vi "Configurator.vi"(9 "CDependencyInspector in":refnum<class "CDependencyInspection.lvclass">, 11 "UIManager in":refnum<class "UIManager.lvclass">) -> (3 "UIManager out":refnum<class "UIManager.lvclass">)   [LabVIEW 2020, in "UserInterface.lvlib" / "UIManager.lvclass"]
uses:
  UIManager/UIManager.lvclass
  DependencyInspection/CItemMatch/TypeDefs/Field.ctl
  DependencyInspection/CItemMatch/TypeDefs/ComparisonType.ctl
  DependencyInspection/CDependencyInspector/CDependencyInspection.lvclass
  ExtensionInterfaces/IConfigurationPage/Event_ParametersRef.ctl
  ExtensionInterfaces/IConfigurationPage/Event_Parameters.ctl
  DependencyInspection/CDependencyInspector/Options.ctl
  DependencyInspection/CDependencyInspector/Options_Export.ctl
  DependencyInspection/CDependencyInspector/Options_Filter.ctl
  DependencyInspection/CItemMatch/CItemMatch.lvclass
  ExtensionInterfaces/IConfigurationPage/IConfigurationPage.lvclass
panel:
  in  "Tab Control":T1(tab)
  in  "Target filter":T4
  in  "Source filter":T4
  in  "Circular deps":bool
  in  "Top level only":bool
  in  "Tests into a separate group":bool
  in  "Path to Check":path
  in  "Exclude instances":bool=TRUE
  in  "Exclude external":bool=TRUE
  in  "Root Path":path
  in  "AND Condition?":bool
  in  "Rules parsers":string(combo)
  in  "Export Rules":bool=TRUE
  in  "Export Dependencies":bool=TRUE
  in  "Exporters":string(combo)
  in  "Export Invalid Dependencies":bool=TRUE
  in  "Export Concessions":bool=TRUE
  in  "Export Undeclared":bool=TRUE
  out "Results":string[][](table)
  in  "Close":bool
  in  "Run":bool
  # "Options"
  # "(780 x 230)"
  # "Options"
  # "(780 x 155)"
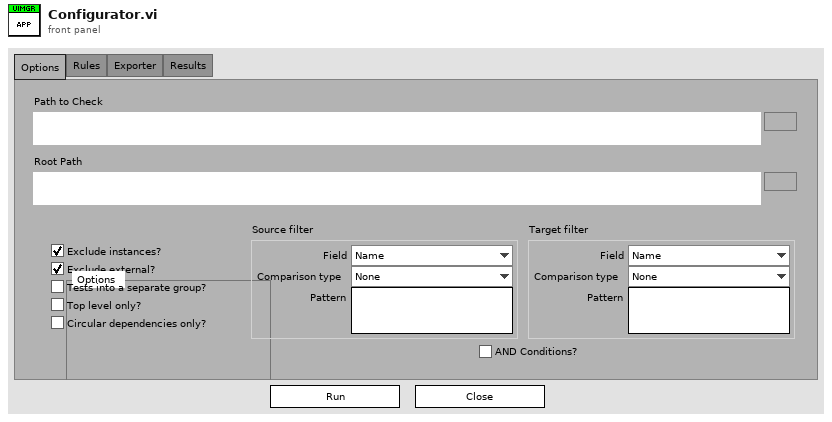
[diagram p1: front panel]
types:
  T1 = enum32{"Options", "Rules", "Exporter", "Results"}
  T2 = typedef "DependencyInspection.lvlib/CItemMatch.lvclass/Field.ctl" = enum16{"Name", "Qualified name", "Path"}
  T3 = typedef "DependencyInspection.lvlib/CItemMatch.lvclass/ComparisonType.ctl" = enum16{"None", "Ends with", "Equals", "Not equal", "Starts with", "Contains", "Matches pattern"}
  T4 = cluster{"Field":T2, "Comparison type":T3, "Pattern":string}
  T5 = typedef "ExtensionInterfaces.lvlib/IConfigurationPage.lvclass/Event_ParametersRef.ctl" = refnum<user-event>
  T6 = typedef "DependencyInspection.lvlib/CDependencyInspection.lvclass/Options.ctl" = cluster{"exclude instances?":bool, "exclude external? (T)":bool, "separate tests?":bool, "top level results only?":bool, "Export options":T7, "Filter options":T8, "quiet?":bool}
  T7 = typedef "DependencyInspection.lvlib/CDependencyInspection.lvclass/Options_Export.ctl" = cluster{"Export rules":bool, "Export dependencies":bool, "Export invalid dependencies":bool, "Export concessions":bool, "Export undeclared":bool}
  T8 = typedef "DependencyInspection.lvlib/CDependencyInspection.lvclass/Options_Filter.ctl" = cluster{"Source filter":refnum<class "CItemMatch.lvclass">, "Target filter":refnum<class "CItemMatch.lvclass">, "AND Condition?":bool}
  T9 = typedef "UserInterface.lvlib/UIManager.lvclass/subReferenceData.ctl" = cluster{"VI Ref":refnum<vi>, "Stop":refnum<user-event>, "Parameters":refnum<user-event>}
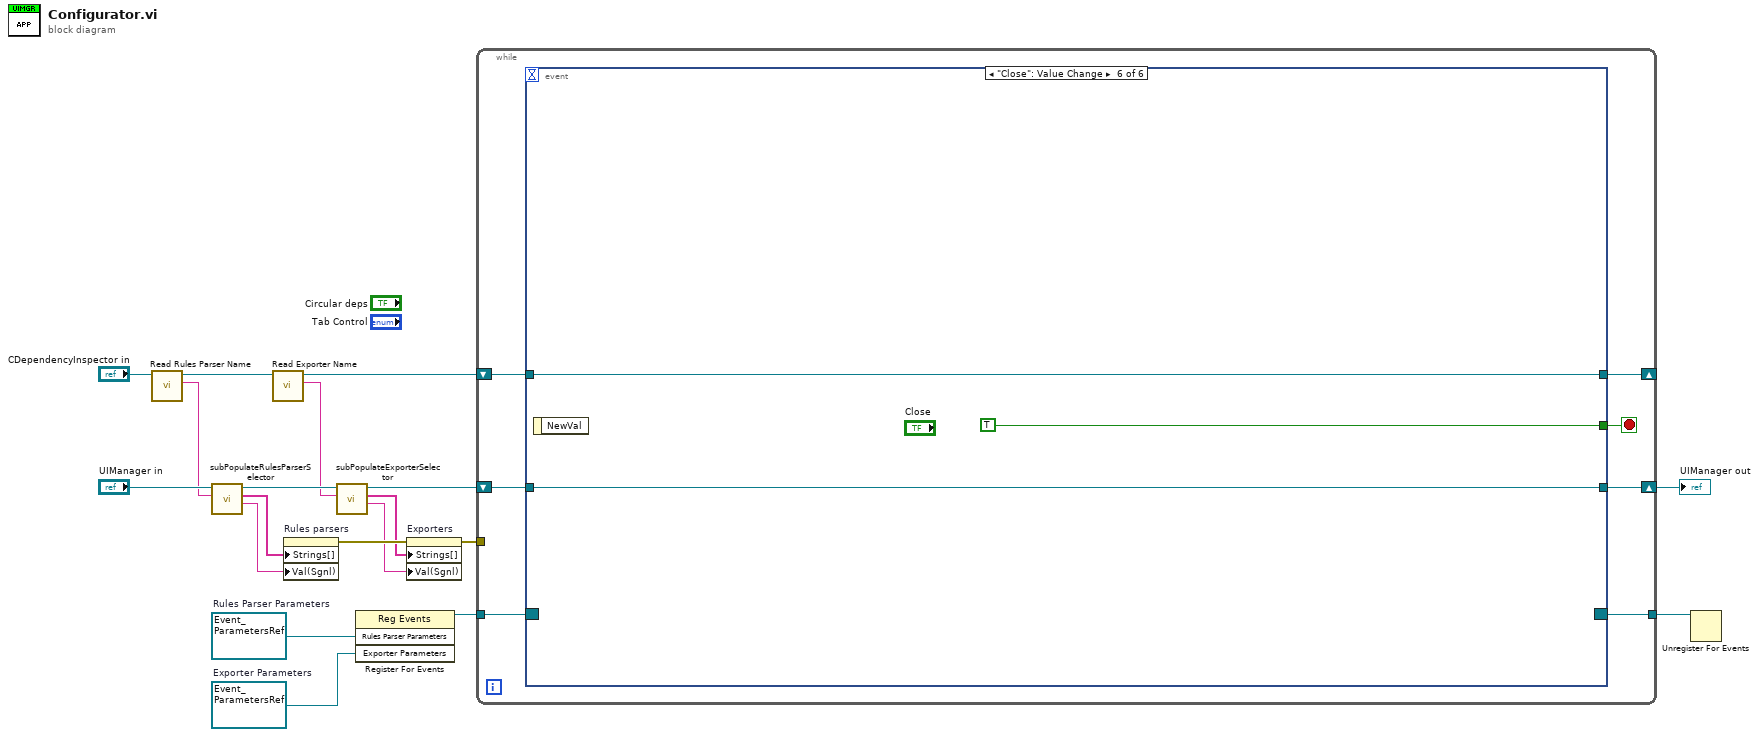
[diagram p0: block diagram]
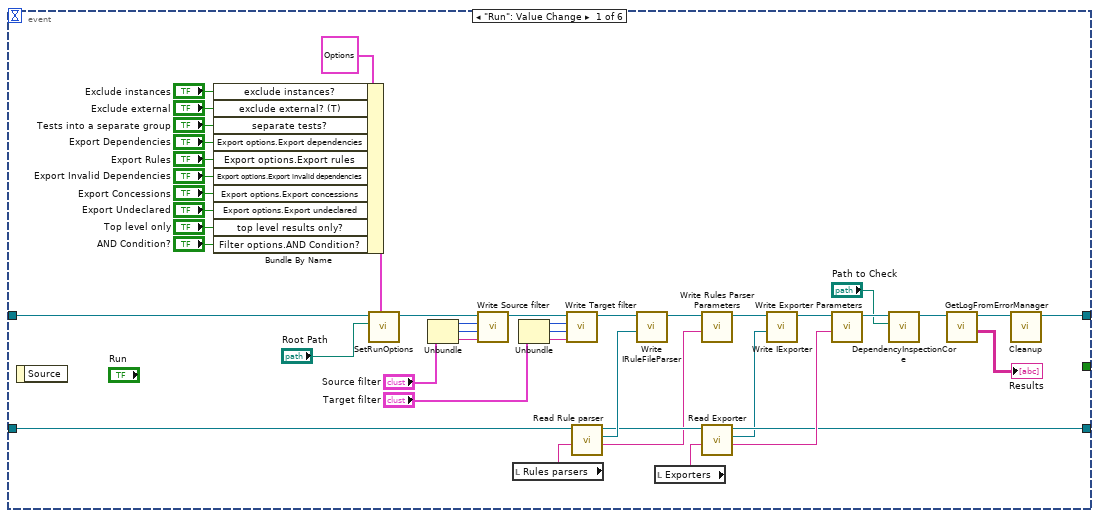
[diagram p2: hidden frame]
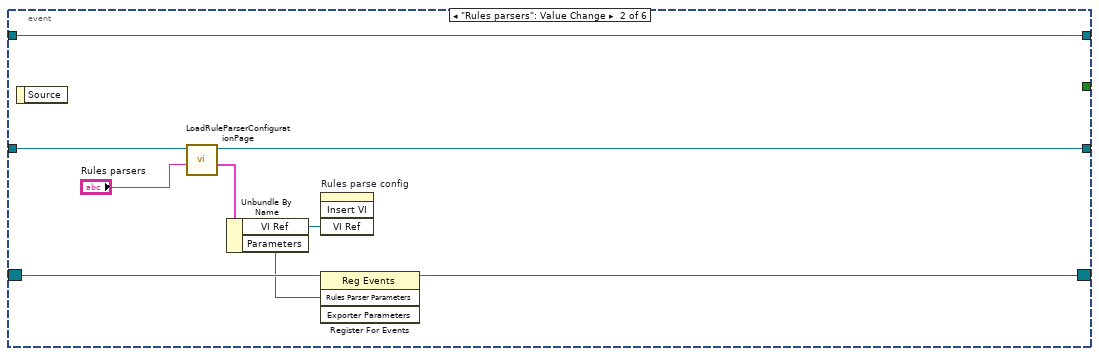
[diagram p3: hidden frame]
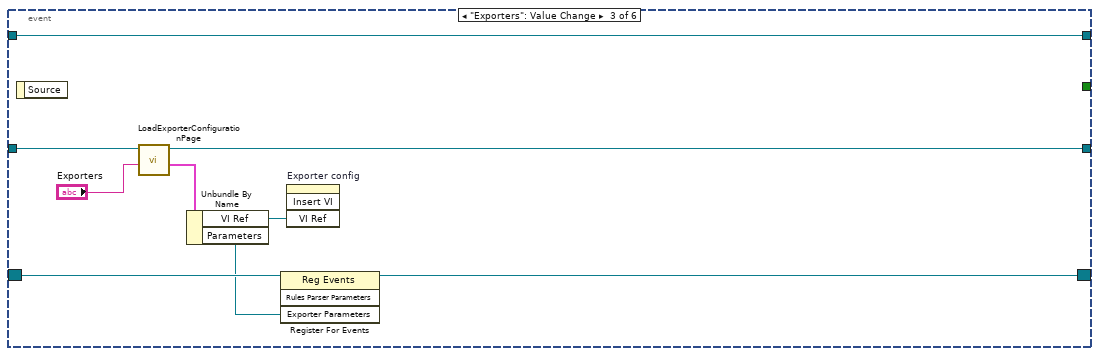
[diagram p4: hidden frame]
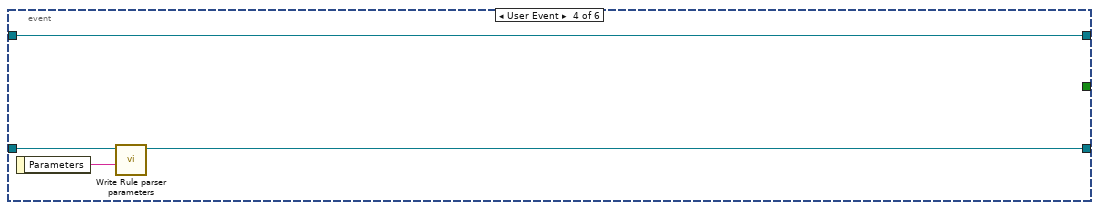
[diagram p5: hidden frame]
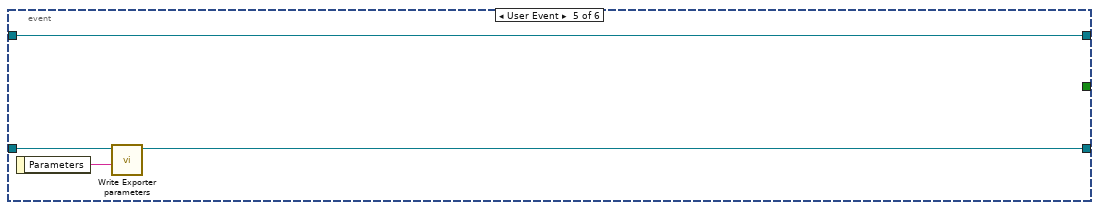
[diagram p6: hidden frame]
diagram:
  w16 = T5 refnum  # Exporter Parameters
  w18 = T5 refnum  # Rules Parser Parameters
  n1 = call-dynamic "Read Rules Parser Name.vi"("CDependencyInspection in"="CDependencyInspector in") -> ("Name"=w7:string, "CDependencyInspection out"=w11:refnum<class "CDependencyInspection.lvclass">)  [unwired: 9 in]
  n2 = call "subPopulateRulesParserSelector.vi"("Selection"=w7, "UIManager in"="UIManager in") -> ("Display name"=w8:string, "Rule parser names"=w9:string[], "UIManager out"=w6:refnum<class "UIManager.lvclass">)  [unwired: 6 in, 1 out]
  n3 = call-dynamic "Read Exporter Name.vi"("CDependencyInspection in"=w11) -> ("Name"=w2:string, "CDependencyInspection out"=w1:refnum<class "CDependencyInspection.lvclass">)  [unwired: 9 in]
  n4 = property on="Rules parsers" class="CmbBox"("Strings[]"=w9, "Val(Sgnl)"=w8) -> (error out=w15:errorcluster)  [unwired: 2 in, 1 out]
  n5 = call "subPopulateExporterSelector.vi"("Selection"=w2, "UIManager in"=w6) -> ("Display name"=w3:string, "Exporter names"=w4:string[], "UIManager out"=w5:refnum<class "UIManager.lvclass">)  [unwired: 6 in, 1 out]
  n6 = register-events(w18, w16) -> (reference out=w19:refnum<event-registration>)  [unwired: 2 in, 1 out]
  n7 = property on="Exporters" class="CmbBox"(error in=w15, "Strings[]"=w4, "Val(Sgnl)"=w3) -> (error out=w14:errorcluster)  [unwired: 1 in, 1 out]
  n8 = while {
    tunnel: w19 -> [w25]
    shift-right: [w23] -> _
    shift-left: w1 -> [w24]
    tunnel: [w22] -> w17
    tunnel: w14 -> [_]
    shift-right: [w20] -> w13
    shift-left: w5 -> [w21]
    stop <- w26 stop-if-true
    n9 = event shown="[5] \"Close\": Value Change" {
      selector: w25 -> [_ w78 w87 _ _ _]
      dyn-events: [_ w77 w86 _ _ _] -> w22
      timeout: _ -> [_ _ _ _ _ _]
      tunnel: [_ _ _ _ _ TRUE] -> w26
      tunnel: w24 -> [w66 w74 w83 w88 w92 w97]
      tunnel: [w42 w74 w83 w88 w92 w97] -> w23
      tunnel: w21 -> [w57 w73 w81 w90 w94 w96]
      tunnel: [w49 w72 w82 w91 w95 w96] -> w20
      event "Run": Value Change {
        n10 = event-data() -> ()  [unwired: 1 in, 1 out]
        n11 = Bundle By Name(cluster=T6 {"exclude instances?"=FALSE, "exclude external? (T)"=TRUE, "separate tests?"=FALSE, "top level results only?"=FALSE, "Export options"={"Export rules"=FALSE, "Export dependencies"=FALSE, "Export invalid dependencies"=FALSE, "Export concessions"=FALSE, "Export undeclared"=FALSE}, "Filter options"={"Source filter"=refnum, "Target filter"=refnum, "AND Condition?"=FALSE}, "quiet?"=FALSE} ("Options"), "exclude instances?"="Exclude instances", "exclude external? (T)"="Exclude external", "separate tests?"="Tests into a separate group", "Export options.Export dependencies"="Export Dependencies", "Export options.Export rules"="Export Rules", "Export options.Export invalid dependencies"="Export Invalid Dependencies", "Export options.Export concessions"="Export Concessions", "Export options.Export undeclared"="Export Undeclared", "top level results only?"="Top level only", "Filter options.AND Condition?"="AND Condition?") -> (w64:T6)
        n12 = call-dynamic "SetRunOptions.vi"("Options"=w64, "Root path"="Root Path", "CDependencyInspection in"=w66) -> ("CDependencyInspection out"=w31:refnum<class "CDependencyInspection.lvclass">)  [unwired: 7 in, 1 out]
        n13 = Unbundle("Source filter") -> ("Field"=w38:T2, "Comparison type"=w37:T3, "Pattern"=w36:string)
        n14 = call-dynamic "Write Source filter.vi"("Filter"=w36, "Comparison type"=w37, "Field"=w38, "CDependencyInspection in"=w31) -> ("CDependencyInspection out"=w40:refnum<class "CDependencyInspection.lvclass">)  [unwired: 7 in]
        n15 = local read "Rules parsers"() -> (w47:string)
        n16 = Unbundle("Target filter") -> ("Field"=w34:T2, "Comparison type"=w33:T3, "Pattern"=w32:string)
        n17 = call-dynamic "Write Target filter.vi"("Filter"=w32, "Comparison type"=w33, "Field"=w34, "CDependencyInspection in"=w40) -> ("CDependencyInspection out"=w30:refnum<class "CDependencyInspection.lvclass">)  [unwired: 7 in]
        n18 = call-dynamic "Read Rule parser.vi"("Selection"=w47, "UIManager in"=w57) -> ("Parameters"=w51:string, "IRuleFileParser.lvclass"=w53:refnum<class "IRuleFileParser.lvclass">, "UIManager out"=w52:refnum<class "UIManager.lvclass">)  [unwired: 5 in, 2 out]
        n19 = call-dynamic "Write IRuleFileParser.vi"("IRuleFileParser"=w53, "CDependencyInspection in"=w30) -> ("CDependencyInspection out"=w56:refnum<class "CDependencyInspection.lvclass">)  [unwired: 9 in]
        n20 = local read "Exporters"() -> (w46:string)
        n21 = call-dynamic "Write Rules Parser Parameters.vi"("Parameters"=w51, "CDependencyInspection in"=w56) -> ("CDependencyInspection out"=w55:refnum<class "CDependencyInspection.lvclass">)  [unwired: 9 in]
        n22 = call-dynamic "Read Exporter.vi"("Selection"=w46, "UIManager in"=w52) -> ("Parameters"=w50:string, "IExporter.lvclass"=w48:refnum<class "IExporter.lvclass">, "UIManager out"=w49:refnum<class "UIManager.lvclass">)  [unwired: 5 in, 2 out]
        n23 = call-dynamic "Write IExporter.vi"("IExporter"=w48, "CDependencyInspection in"=w55) -> ("CDependencyInspection out"=w54:refnum<class "CDependencyInspection.lvclass">)  [unwired: 9 in]
        n24 = call-dynamic "Write Exporter Parameters.vi"("Parameters"=w50, "CDependencyInspection in"=w54) -> ("CDependencyInspection out"=w29:refnum<class "CDependencyInspection.lvclass">)  [unwired: 9 in]
        n25 = call-dynamic "DependencyInspectionCore.vi"("Path to Check"="Path to Check", "CDependencyInspection in"=w29) -> ("CDependencyInspection out"=w28:refnum<class "CDependencyInspection.lvclass">)  [unwired: 9 in]
        n26 = call-dynamic "GetLogFromErrorManager.vi"("CDependencyInspection in"=w28) -> ("Log results"=→"Results":string[][], "CDependencyInspection out"=w43:refnum<class "CDependencyInspection.lvclass">)  [unwired: 8 in, 1 out]
        n27 = call-dynamic "Cleanup.vi"("CDependencyInspection in"=w43) -> ("CDependencyInspection out"=w42:refnum<class "CDependencyInspection.lvclass">)  [unwired: 9 in, 1 out]
      }
      event "Rules parsers": Value Change {
        n28 = event-data() -> ()  [unwired: 1 in, 1 out]
        n29 = call-dynamic "LoadRuleParserConfigurationPage.vi"("Selection"="Rules parsers", "UIManager in"=w73) -> ("References"=w70:T9, "UIManager out"=w72:refnum<class "UIManager.lvclass">)  [unwired: 7 in, 1 out]
        n30 = Unbundle By Name(w70) -> ("VI Ref"=w76:refnum<vi>, "Parameters"=w75:refnum<user-event>)
        n31 = invoke on="Rules parse config" class="SubPnl" method="Insert VI"("VI Ref"=w76) -> ()  [unwired: 3 in, 4 out]
        n32 = register-events(reference=w78, w75) -> (reference out=w77:refnum<event-registration>)  [unwired: 2 in, 1 out]
      }
      event "Exporters": Value Change {
        n33 = event-data() -> ()  [unwired: 1 in, 1 out]
        n34 = call-dynamic "LoadExporterConfigurationPage.vi"("Selection"="Exporters", "UIManager in"=w81) -> ("References"=w79:T9, "UIManager out"=w82:refnum<class "UIManager.lvclass">)  [unwired: 7 in, 1 out]
        n35 = Unbundle By Name(w79) -> ("VI Ref"=w85:refnum<vi>, "Parameters"=w84:refnum<user-event>)
        n36 = register-events(reference=w87, w84) -> (reference out=w86:refnum<event-registration>)  [unwired: 2 in, 1 out]
        n37 = invoke on="Exporter config" class="SubPnl" method="Insert VI"("VI Ref"=w85) -> ()  [unwired: 3 in, 4 out]
      }
      event User Event {
        n38 = event-data() -> ("Parameters"=w89:string)  [unwired: 1 in]
        n39 = call-dynamic "Write Rule parser parameters.vi"("Parameters"=w89, "UIManager in"=w90) -> ("UIManager out"=w91:refnum<class "UIManager.lvclass">)  [unwired: 9 in]
      }
      event User Event {
        n40 = event-data() -> ("Parameters"=w93:string)  [unwired: 1 in]
        n41 = call-dynamic "Write Exporter parameters.vi"("Parameters"=w93, "UIManager in"=w94) -> ("UIManager out"=w95:refnum<class "UIManager.lvclass">)  [unwired: 9 in]
      }
      event "Close": Value Change {
        n42 = event-data() -> ()  [unwired: 1 in, 1 out]
      }
    }
  }
  "UIManager out" <- w13
  n43 = Unregister For Events(event registration refnum=w17) -> ()  [unwired: 1 in, 1 out]
